vi "DetectTrajectoryCollision.vi"(4 "ball":dbl[](array[numeric]), 6 "our_robots":T1[](array[typedef]), 7 "Robot in":T1, 8 "Goal":dbl[](array[numeric]), 9 "Initial State":dbl[](array[numeric]), 10 "Last Path":dbl[][](array[numeric]), 11 "enemy_robots":T1[](array[typedef])) -> (2 "Collision":bool)   [LabVIEW 2018]
uses:
  Core/AI Robot.ctl
  Intel/Functions Enum.ctl
  Intel/AttackerStates.ctl
  PathDests.ctl
  PathDest.ctl
  <vilib>/Analysis/NI_AALPro.lvlib
  <vilib>/Analysis/_algsub.llb/Real Vector Norm.vi
panel:
  out "Is there colision?":bool
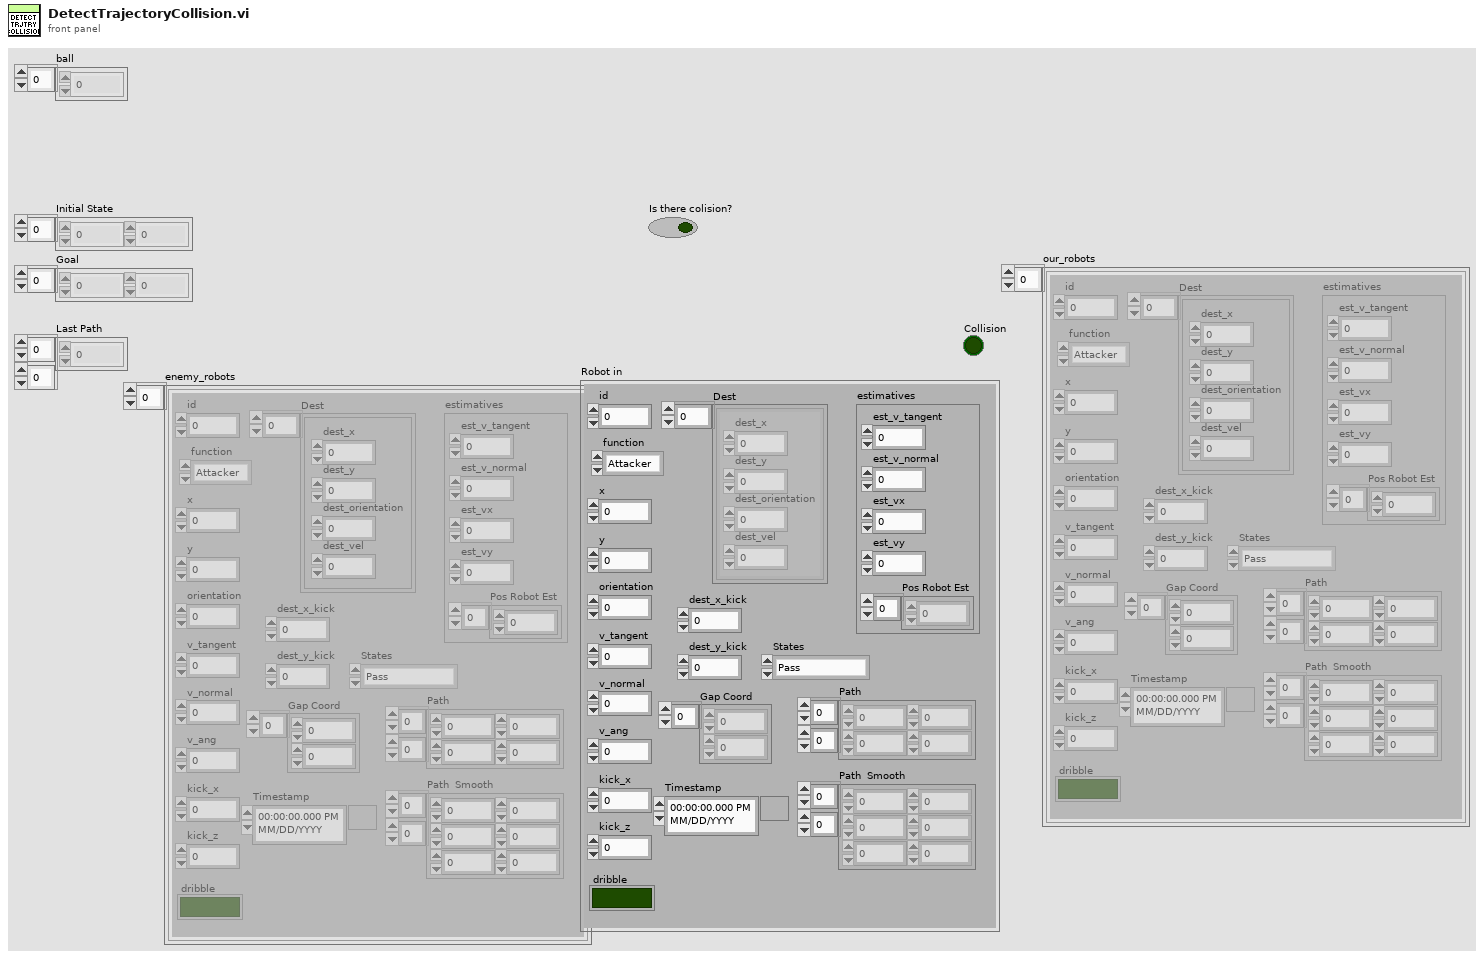
[diagram p1: front panel]
types:
  T1 = typedef "AI Robot.ctl" = cluster{"id":u32, "function":T2, "x":dbl, "y":dbl, "orientation":dbl, "v_tangent":dbl, "v_normal":dbl, "v_ang":dbl, "kick_x":dbl, "kick_z":dbl, "dribble":bool, "Timestamp":timestamp, "estimatives":cluster{"est_v_tangent":dbl, "est_v_normal":dbl, "est_vx":dbl, "est_vy":dbl, "Pos Robot Est":dbl[]}, "dest_x_kick":dbl, "dest_y_kick":dbl, "Gap Coord":dbl[], "States":T3, "Path ":dbl[][], "Path  Smooth":dbl[][], "Dest":T4}
  T2 = typedef "Functions Enum.ctl" = enum16{"Attacker", "Goalie", "Defender", "Striker", "Goto 0", "Dummy", "Kicker", "ZigZag"}
  T3 = typedef "AttackerStates.ctl" = enum16{"Pass", "GoToTangent", "BallGetting", "GoToKick", "Rotate anti-clockwise", "Rotate Clockwise", ""}
  T4 = typedef "PathDests.ctl" = T5[]
  T5 = typedef "PathDest.ctl" = cluster{"dest_x":dbl, "dest_y":dbl, "dest_orientation":dbl, "dest_vel":dbl}
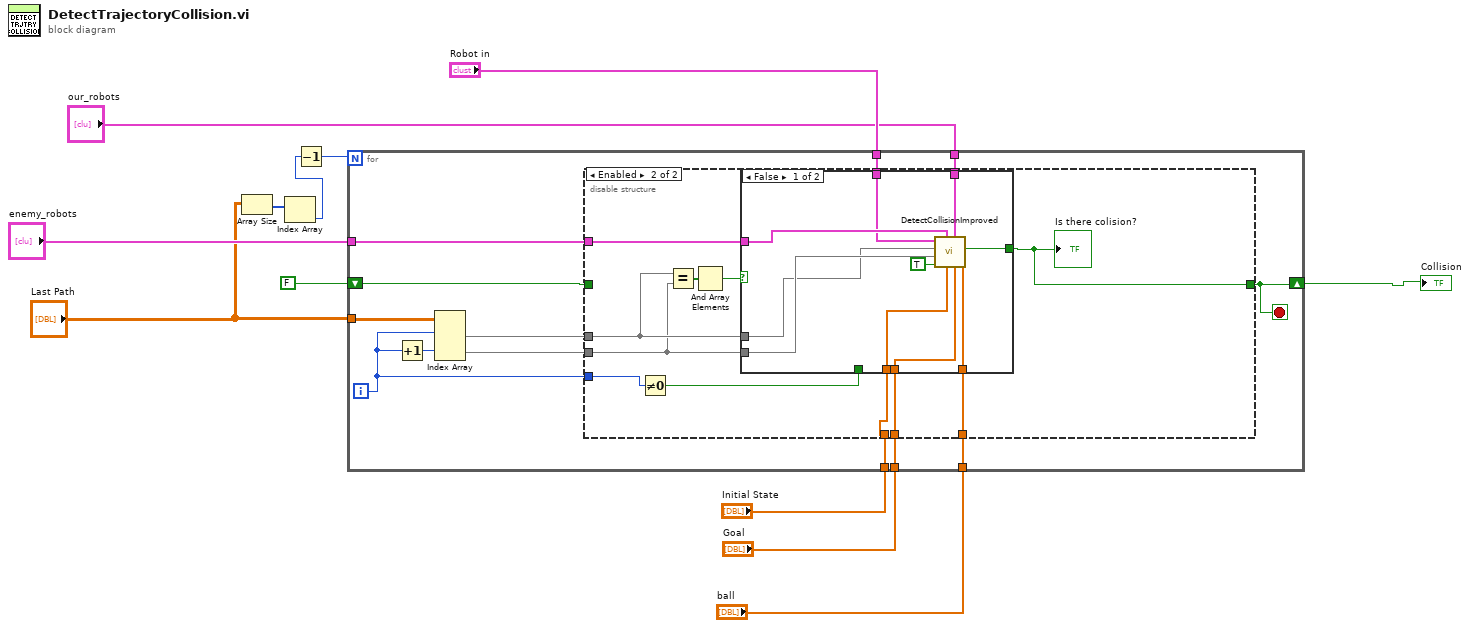
[diagram p0: block diagram]
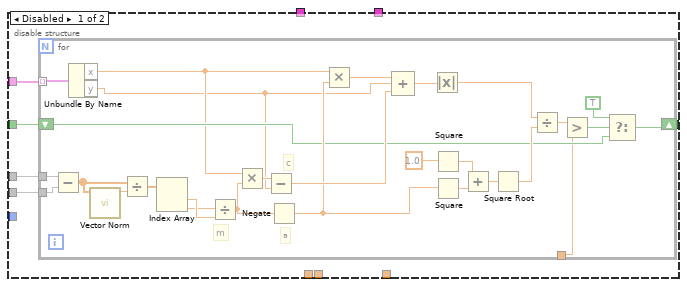
[diagram p2: hidden frame]
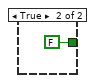
[diagram p3: hidden frame]
diagram:
  n1 = Array Size(array="Last Path") -> (size(s)=w9:i32[])
  n2 = Index Array(array=w9) -> (element=w4:i32)  [unwired: 1 in]
  n3 = Decrement(x=w4) -> (x-1=w5:i32)
  n4 = for {
    N: w5 -> [_]
    tunnel: "enemy_robots" -> [w25]
    tunnel: "Last Path" -> [w24]
    shift-right: [w20] -> w3
    shift-left: FALSE -> [w21]
    tunnel: "Robot in" -> [w17]
    tunnel: "Initial State" -> [w16]
    tunnel: "Goal" -> [w15]
    tunnel: "our_robots" -> [w14]
    tunnel: "ball" -> [w13]
    i -> [w18]
    stop <- w20 stop-if-true
    n5 = Increment(x=w18) -> (x+1=w19:i32)
    n6 = Index Array(array=w24, index (row) #1=w18, index (row) #2=w19) -> (element #1=w23:dbl[], element #2=w22:dbl[])  [unwired: 2 in]
    n7 = disable-structure shown="Enabled" {
      disable-tunnel: w25 -> [w30 w69]
      disable-tunnel: w23 -> [w29 w64]
      disable-tunnel: w22 -> [w28 w63]
      disable-tunnel: w21 -> [w27 _]
      disable-tunnel: [w26 w65] -> w20
      disable-tunnel: w18 -> [_ w71]
      disable-tunnel: w17 -> [_ w70]
      disable-tunnel: w16 -> [_ w67]
      disable-tunnel: w15 -> [_ w66]
      disable-tunnel: w14 -> [_ w60]
      disable-tunnel: w13 -> [_ w59]
      frame Disabled {
        n8 = for {
          tunnel: w30 -> [w51] mode=indexing
          tunnel: w29 -> [w58]
          tunnel: w28 -> [w57]
          tunnel: _ -> [w31]
          shift-right: [w38] -> w26
          shift-left: w27 -> [w36]
          # "c"
          # "a"
          # "m"
          n9 = Subtract(x=w58, y=w57) -> (x-y=w55:dbl[])
          n10 = Unbundle By Name(w51) -> ("x"=w33:dbl, "y"=w32:dbl)
          n11 = call-poly <vilib>:"Vector Norm.vi"("Input Vector"=w55) -> ("norm"=w56:dbl)  [unwired: 9 in, 1 out]
          n12 = Divide(x=w55, y=w56) -> (x/y=w54:dbl[])
          n13 = Index Array(array=w54) -> (element #1=w53:dbl, element #2=w34:dbl)  [unwired: 2 in]
          n14 = Divide(x=w34, y=w53) -> (x/y=w52:dbl)
          n15 = Multiply(x=w33, y=w52) -> (x*y=w35:dbl)
          n16 = Subtract(x=w35, y=w32) -> (x-y=w49:dbl)
          n17 = Negate(x=w52) -> (-x=w45:dbl)
          n18 = Multiply(x=w33, y=w45) -> (x*y=w50:dbl)
          n19 = Compound Arithmetic op=ADD(w50, w32, w49) -> (w48:dbl)
          n20 = Absolute Value(x=w48) -> (abs(x)=w42:dbl)
          n21 = Square(x=1.0) -> (x^2=w47:dbl)
          n22 = Square(x=w45) -> (x^2=w46:dbl)
          n23 = Add(x=w47, y=w46) -> (x+y=w43:dbl)
          n24 = Square Root(x=w43) -> (sqrt(x)=w41:dbl)
          n25 = Divide(x=w42, y=w41) -> (x/y=w40:dbl)
          n26 = Greater?(x=w40, y=w31) -> (0:w39:bool)
          n27 = Select(t=TRUE, s=w39, f=w36) -> (s? t:f=w38:bool)
        }
      }
      frame Enabled {
        n28 = Not Equal To 0?(x=w71) -> (x != 0?=w68:bool)
        n29 = Equal?(x=w64, y=w63) -> (x = y?=w62:bool[])
        n30 = And Array Elements(Boolean array=w62) -> (logical AND=w61:bool)
        n31 = case shown="False" w61 {
          tunnel: w70 -> [w75 _]
          tunnel: w69 -> [w76 _]
          tunnel: w63 -> [w81 _]
          tunnel: w64 -> [w80 _]
          tunnel: w68 -> [_ _]
          tunnel: w67 -> [w79 _]
          tunnel: w66 -> [w74 _]
          tunnel: [w77 FALSE ("Is there colision?")] -> w65
          tunnel: w60 -> [w73 _]
          tunnel: w59 -> [w72 _]
          frame False {
            n32 = call "DetectCollisionImproved.vi"("ball"=w72, "Goal"=w74, "our_robots"=w73, "Initial State"=w79, "enemy_robots"=w76, "Is not first robot?"=TRUE, "element being analyzed"=w81, "element already in path"=w80, "Robot in"=w75) -> ("Is there colision?"=w77:bool)  [unwired: 2 in]
          }
          frame True {
          }
        }
        "Is there colision?" <- w65
      }
    }
  }
  "Collision" <- w3
